vi "Draw Ellipse.vi"(10 "picture":picture, 11 "Ellipse":T1 {"Minor Axis"."Point 2"."Y" format="%.2f"; "Minor Axis"."Point 2"."X" format="%.2f"; "Minor Axis"."Point 1"."Y" format="%.2f"; "Minor Axis"."Point 1"."X" format="%.2f"; "Major Axis"."Point 2"."Y" format="%.2f"; "Major Axis"."Point 2"."X" format="%.2f"; "Major Axis"."Point 1"."Y" format="%.2f"; "Major Axis"."Point 1"."X" format="%.2f"; "Center"."Y" format="%.2f"; "Center"."X" format="%.2f"}) -> (3 "new picture":picture)   [LabVIEW 2013]
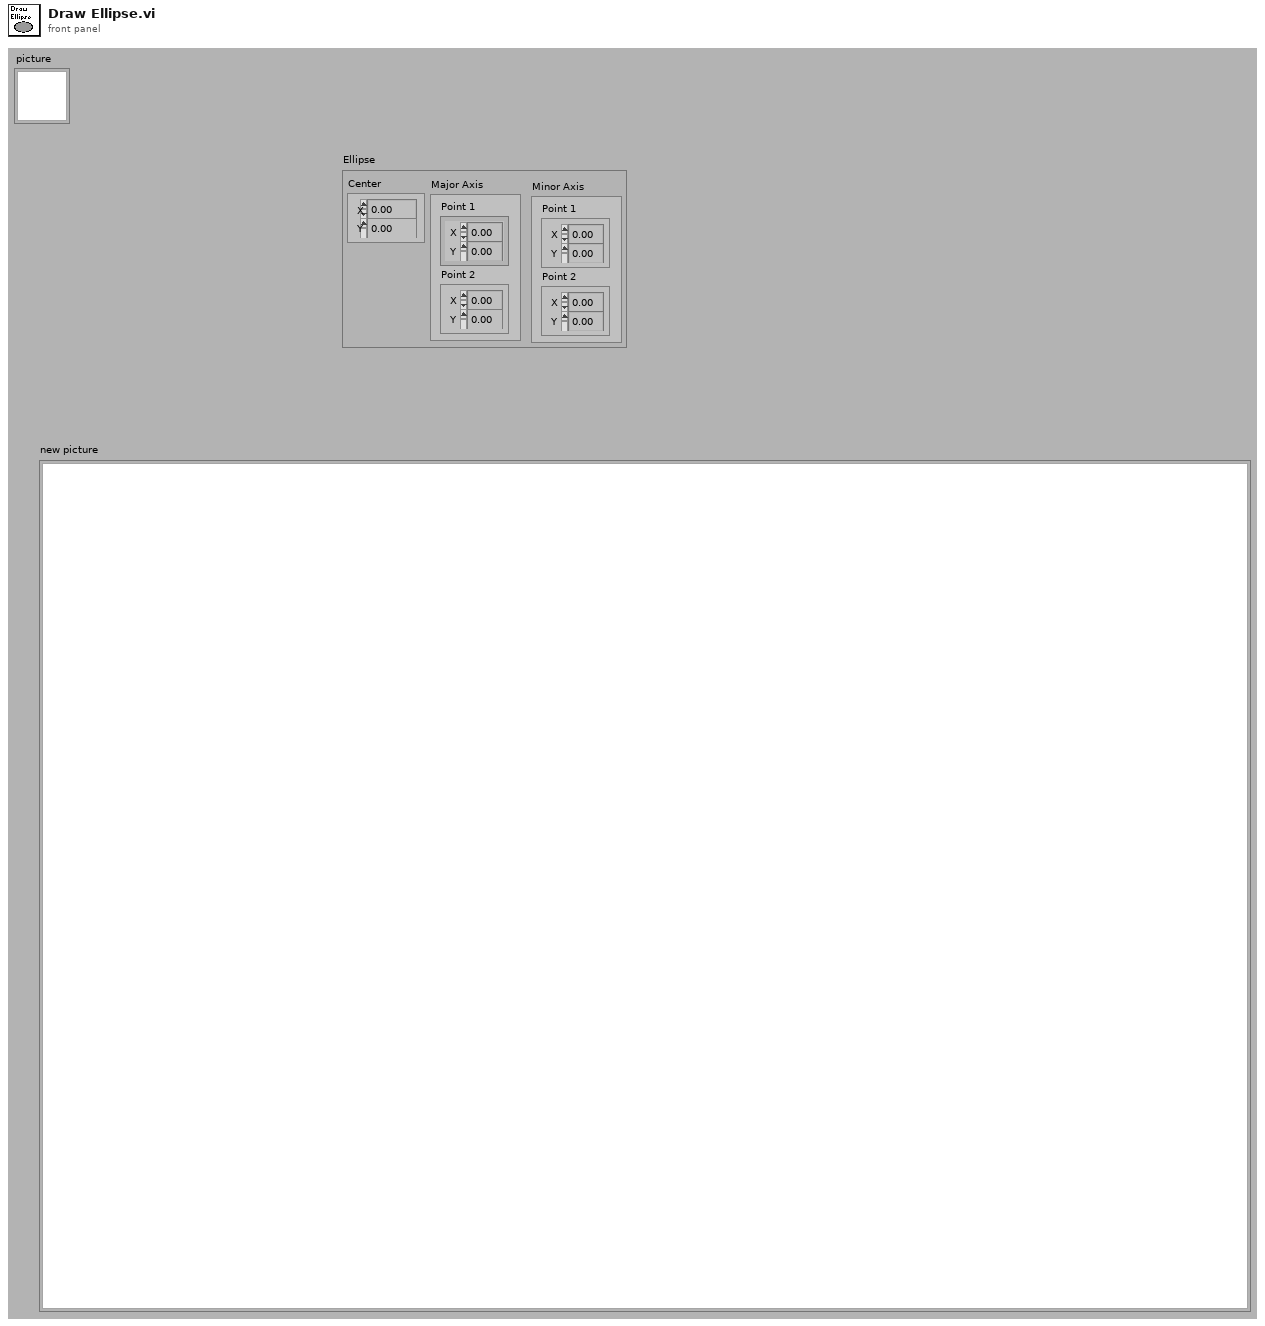
[diagram p1: front panel]
types:
  T1 = cluster{"Center":cluster{"X":sgl, "Y":sgl}, "Major Axis":cluster{"Point 1":cluster{"X":sgl, "Y":sgl}, "Point 2":cluster{"X":sgl, "Y":sgl}}, "Minor Axis":cluster{"Point 1":cluster{"X":sgl, "Y":sgl}, "Point 2":cluster{"X":sgl, "Y":sgl}}}
  T2 = cluster{"Width":u16, "Style":enum32{"Solid", "Dash", "Dot", "DashDot", "DashDotDot"}}
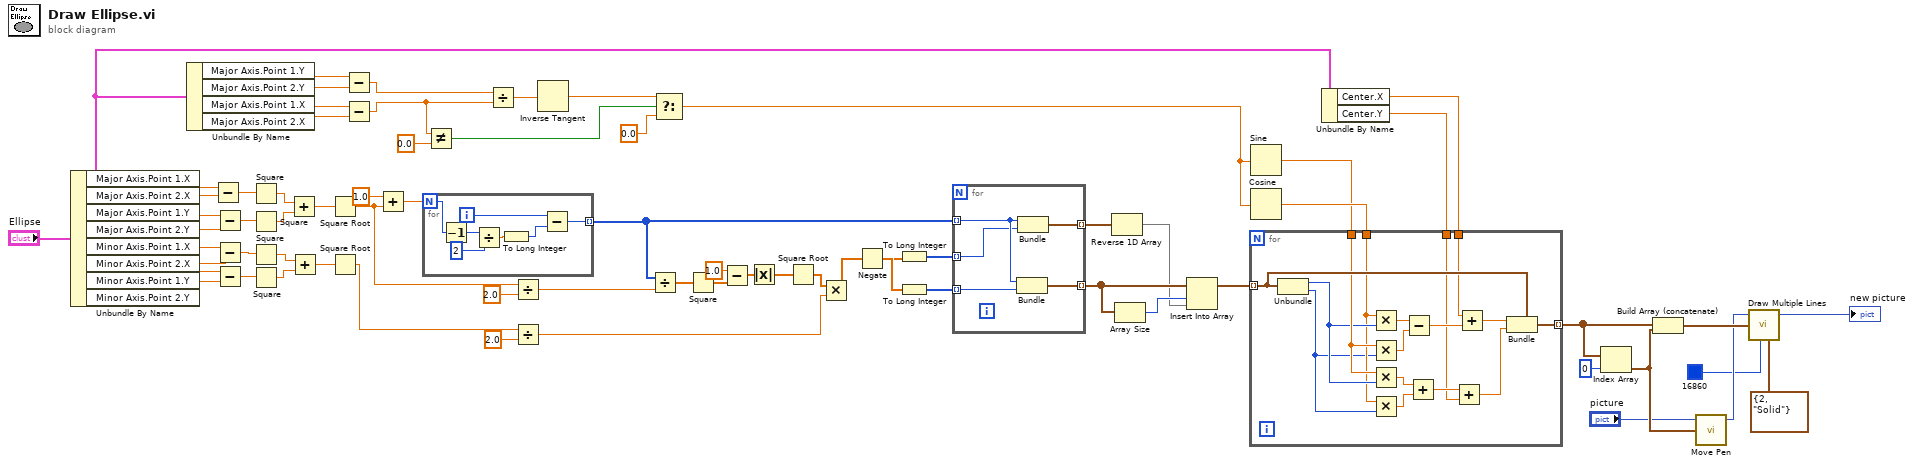
[diagram p0: block diagram]
diagram:
  n1 = Unbundle By Name("Ellipse") -> ("Major Axis.Point 1.X"=w67:sgl, "Major Axis.Point 2.X"=w68:sgl, "Major Axis.Point 1.Y"=w66:sgl, "Major Axis.Point 2.Y"=w65:sgl, "Minor Axis.Point 1.X"=w36:sgl, "Minor Axis.Point 2.X"=w64:sgl, "Minor Axis.Point 1.Y"=w63:sgl, "Minor Axis.Point 2.Y"=w62:sgl)
  n2 = Unbundle By Name("Ellipse") -> ("Major Axis.Point 1.Y"=w35:sgl, "Major Axis.Point 2.Y"=w34:sgl, "Major Axis.Point 1.X"=w33:sgl, "Major Axis.Point 2.X"=w32:sgl)
  n3 = Subtract(x=w67, y=w68) -> (x-y=w61:sgl)
  n4 = Subtract(x=w66, y=w65) -> (x-y=w60:sgl)
  n5 = Subtract(x=w36, y=w64) -> (x-y=w59:sgl)
  n6 = Subtract(x=w63, y=w62) -> (x-y=w58:sgl)
  n7 = Square(x=w61) -> (x^2=w57:sgl)
  n8 = Square(x=w60) -> (x^2=w55:sgl)
  n9 = Square(x=w59) -> (x^2=w56:sgl)
  n10 = Square(x=w58) -> (x^2=w54:sgl)
  n11 = Add(x=w57, y=w55) -> (x+y=w53:sgl)
  n12 = Add(x=w56, y=w54) -> (x+y=w52:sgl)
  n13 = Square Root(x=w53) -> (sqrt(x)=w16:sgl)
  n14 = Square Root(x=w52) -> (sqrt(x)=w20:sgl)
  n15 = Subtract(x=w35, y=w34) -> (x-y=w31:sgl)
  n16 = Subtract(x=w33, y=w32) -> (x-y=w13:sgl)
  n17 = Add(x=sgl 1.0, y=w16) -> (x+y=w50:sgl)
  n18 = for {
    N: w50 -> [w75]
    tunnel: [w71] -> w45 mode=indexing
    i -> [w72]
    n19 = Decrement(x=w75) -> (x-1=w74:i32)
    n20 = Divide(x=w74, y=2) -> (x/y=w70:dbl)
    n21 = To Long Integer(number=w70) -> (32bit integer=w69:i32)
    n22 = Subtract(x=w72, y=w69) -> (x-y=w71:i32)
  }
  n23 = Not Equal?(x=w13, y=sgl 0.0) -> (x != y?=w10:bool)
  n24 = Divide(x=w31, y=w13) -> (x/y=w30:sgl)
  n25 = Divide(x=w16, y=sgl 2.0) -> (x/y=w15:sgl)
  n26 = Divide(x=w20, y=sgl 2.0) -> (x/y=w19:sgl)
  n27 = Inverse Tangent(1:w30) -> (0:w11:sgl)
  n28 = Divide(x=w45, y=w15) -> (x/y=w49:sgl[])
  n29 = Select(t=w11, s=w10, f=sgl 0.0) -> (s? t:f=w6:sgl)
  n30 = Square(x=w49) -> (x^2=w47:sgl[])
  n31 = Subtract(x=1.0, y=w47) -> (x-y=w2:dbl[])
  n32 = Absolute Value(x=w2) -> (abs(x)=w3:dbl[])
  n33 = Square Root(x=w3) -> (sqrt(x)=w46:dbl[])
  n34 = Multiply(x=w46, y=w19) -> (x*y=w44:dbl[])
  n35 = Negate(x=w44) -> (-x=w43:dbl[])
  n36 = To Long Integer(number=w43) -> (32bit integer=w42:i32[])
  n37 = To Long Integer(number=w44) -> (32bit integer=w41:i32[])
  n38 = for {
    tunnel: w45 -> [w80] mode=indexing
    tunnel: w42 -> [w79] mode=indexing
    tunnel: w41 -> [w78] mode=indexing
    tunnel: [w77] -> w40 mode=indexing
    tunnel: [w76] -> w39 mode=indexing
    n39 = Bundle(w80, w78) -> (w76:cluster{i32, i32})  [unwired: 1 in]
    n40 = Bundle(w80, w79) -> (w77:cluster{i32, i32})  [unwired: 1 in]
  }
  n41 = Reverse 1D Array(array=w40) -> (reversed array=w37:cluster{i32, i32}[])
  n42 = Array Size(array=w39) -> (size(s)=w38:i32)
  n43 = Insert Into Array(array=w39, index=w38, new element=w37) -> (w5:cluster{i32, i32}[])
  n44 = Sine(x=w6) -> (sin(x)=w7:sgl)
  n45 = Cosine(x=w6) -> (cos(x)=w8:sgl)
  n46 = Unbundle By Name("Ellipse") -> ("Center.X"=w29:sgl, "Center.Y"=w28:sgl)
  n47 = for {
    tunnel: w5 -> [w96] mode=indexing
    tunnel: w8 -> [w88]
    tunnel: w7 -> [w90]
    tunnel: w29 -> [w92]
    tunnel: w28 -> [w83]
    tunnel: [w81] -> w4 mode=indexing
    n48 = Unbundle(w96) -> (w89:i32, w87:i32)
    n49 = Multiply(x=w88, y=w89) -> (x*y=w95:sgl)
    n50 = Multiply(x=w90, y=w87) -> (x*y=w94:sgl)
    n51 = Multiply(x=w90, y=w89) -> (x*y=w86:sgl)
    n52 = Multiply(x=w88, y=w87) -> (x*y=w84:sgl)
    n53 = Subtract(x=w95, y=w94) -> (x-y=w93:sgl)
    n54 = Add(x=w86, y=w84) -> (x+y=w85:sgl)
    n55 = Add(x=w85, y=w83) -> (x+y=w82:sgl)
    n56 = Add(x=w92, y=w93) -> (x+y=w91:sgl)
    n57 = Bundle(cluster=w96, w91, w82) -> (w81:cluster{i32, i32})
  }
  n58 = Index Array(array=w4, index=0) -> (element=w25:cluster{i32, i32})
  n59 = Build Array (concatenate)(w4, w25) -> (w27:cluster{i32, i32}[])
  n60 = call <vilib>:"Move Pen.vi"("new position"=w25, "picture"="picture") -> ("new picture"=w24:picture)  [unwired: 3 in]
  n61 = call <vilib>:"Draw Multiple Lines.vi"("picture"=w24, "line endpoints"=w27, "color(black)"=u32 16860, "pen"=T2 {"Width"=2, "Style"=enum."Solid"}) -> ("new picture"=→"new picture":picture)  [unwired: 5 in]
